vi "getFilterStatus.vi"(8 "error in (no error)":errorcluster, 9 "Filter":T1, 10 "Measurement Function":T2, 11 "Electrometer in":refnum<class "Electrometer.lvclass">) -> (0 "error out":errorcluster, 1 "queryOK?":bool, 2 "Active?":bool, 3 "Electrometer out":refnum<class "Electrometer.lvclass">)   [LabVIEW 2016, in "Electrometer.lvclass"]
uses:
  Electrometer.lvclass
  Modes.ctl
  filterType.ctl
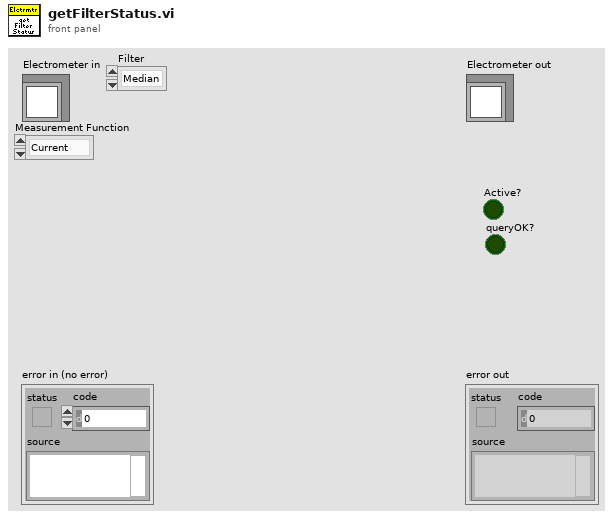
[diagram p1: front panel]
types:
  T1 = typedef "Electrometer.lvclass/filterType.ctl" = enum16{"Median", "Average"}
  T2 = typedef "Electrometer.lvclass/Modes.ctl" = enum16{"Current", "Charge", "Voltage", "Resistance"}
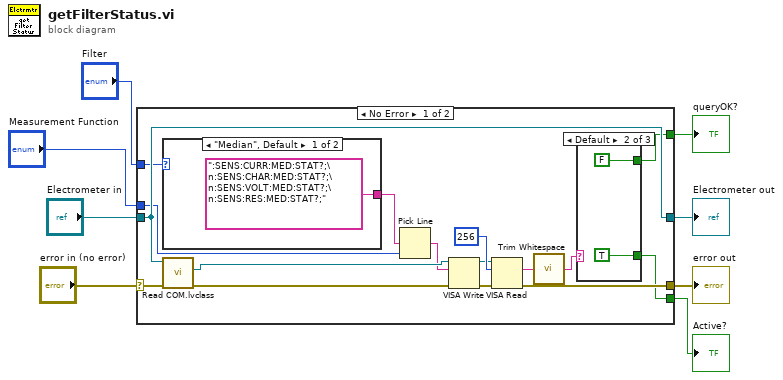
[diagram p0: block diagram]
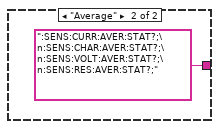
[diagram p2: hidden frame]
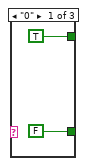
[diagram p3: hidden frame]
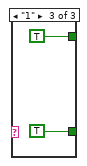
[diagram p4: hidden frame]
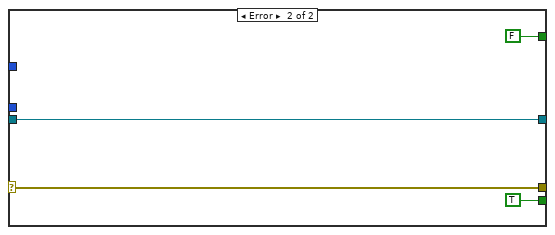
[diagram p5: hidden frame]
diagram:
  n1 = case shown="No Error" "error in (no error)" {
    selector: "error in (no error)" -> [w17 w36]
    tunnel: [w16 w36] -> w7
    tunnel: [w15 w35] -> w5
    tunnel: "Electrometer in" -> [w15 w35]
    tunnel: "Measurement Function" -> [w14 _]
    tunnel: "Filter" -> [w13 _]
    tunnel: [w12 TRUE] -> w2
    tunnel: [w11 FALSE] -> w1
    frame No Error {
      n2 = case shown="\"Median\", Default" w13 {
        tunnel: [":SENS:CURR:MED:STAT?;\n:SENS:CHAR:MED:STAT?;\n:SENS:VOLT:MED:STAT?;\n:SENS:RES:MED:STAT?;" ":SENS:CURR:AVER:STAT?;\n:SENS:CHAR:AVER:STAT?;\n:SENS:VOLT:AVER:STAT?;\n:SENS:RES:AVER:STAT?;"] -> w23
        frame "Median", Default {
        }
        frame "Average" {
        }
      }
      n3 = call "Read COM.lvclass.vi"("error in (no error)"=w17, "Electrometer in"=w15) -> ("error out"=w19:errorcluster, "VISA"=w24:refnum<visa-resource-name>)  [unwired: 7 in, 1 out]
      n4 = Pick Line(multi-line string=w23, line index=w14) -> (output string=w18:string)  [unwired: 1 in]
      n5 = VISA Write(VISA resource name=w24, write buffer=w18, error in (no error)=w19) -> (VISA resource name out=w21:refnum<visa-resource-name>, error out=w20:errorcluster)  [unwired: 1 out]
      n6 = VISA Read(VISA resource name=w21, byte count=u32 256, error in (no error)=w20) -> (read buffer=w10:string, error out=w16:errorcluster)  [unwired: 2 out]
      n7 = call <vilib>:"Trim Whitespace.vi"("string"=w10) -> ("trimmed string"=w9:string)  [unwired: 1 in]
      n8 = case shown="Default" w9 {
        tunnel: [TRUE FALSE TRUE] -> w11
        tunnel: [FALSE TRUE TRUE] -> w12
        frame "0" {
        }
        frame Default {
        }
        frame "1" {
        }
      }
    }
    frame Error {
    }
  }
  "error out" <- w7
  "Electrometer out" <- w5
  "Active?" <- w2
  "queryOK?" <- w1
